vi "from string.vi"(8 "error in":errorcluster, 9 "data":string, 10 "version":string, 11 "Profibus Module configuration in":refnum<class "Profibus Module configuration.lvclass">) -> (0 "error out":errorcluster, 3 "Profibus Module configuration out":refnum<class "Profibus Module configuration.lvclass">)   [LabVIEW 2013, in "Profibus Module configuration.lvclass"]
doc: "Provides an interface for loading a module configuration from a file or other serialized data source. It is recommended that all children of this class store data in two sets--data required for its own initialization, and any data required for parent initialization--and that each implementation uses the <b>Call Parent Method</b> primitive to de-serialize parent information. As a result, it is expected that every module configuration class calls <b>component configuration.lvclass:From String.vi</b>."
uses:
  Profibus Module configuration.lvclass
  <vilib>/NI/Tag Bus Module Framework/module configuration/TBM module configuration.lvclass
  channel/Profibus channel.lvclass
  endianness setting.ctl
  <vilib>/NI/Tag Bus Module Framework/channel/TBM channel.lvclass
  error throw specification.ctl
  slave diagnostic configuration.ctl
  <vilib>/NI/Configuration Framework/serializable configuration/NISE_CEF_serializable configuration.lvclass
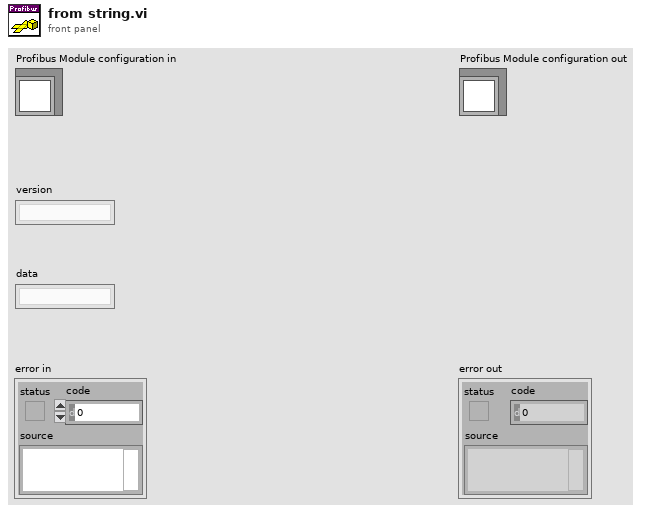
[diagram p1: front panel]
types:
  T1 = typedef "Profibus Module configuration.lvclass/slave diagnostic configuration.ctl" = cluster{"slave":i8, "report":bool, "channel":refnum<class "TBM channel.lvclass">, "error specs":T2[]}
  T2 = typedef "Profibus Module configuration.lvclass/error throw specification.ctl" = cluster{"byte":i32, "bit":i32, "inverted?":bool, "error":i32}
  T3 = typedef "Profibus Module configuration.lvclass/endianness setting.ctl" = cluster{"slave":i8, "big endian":bool}
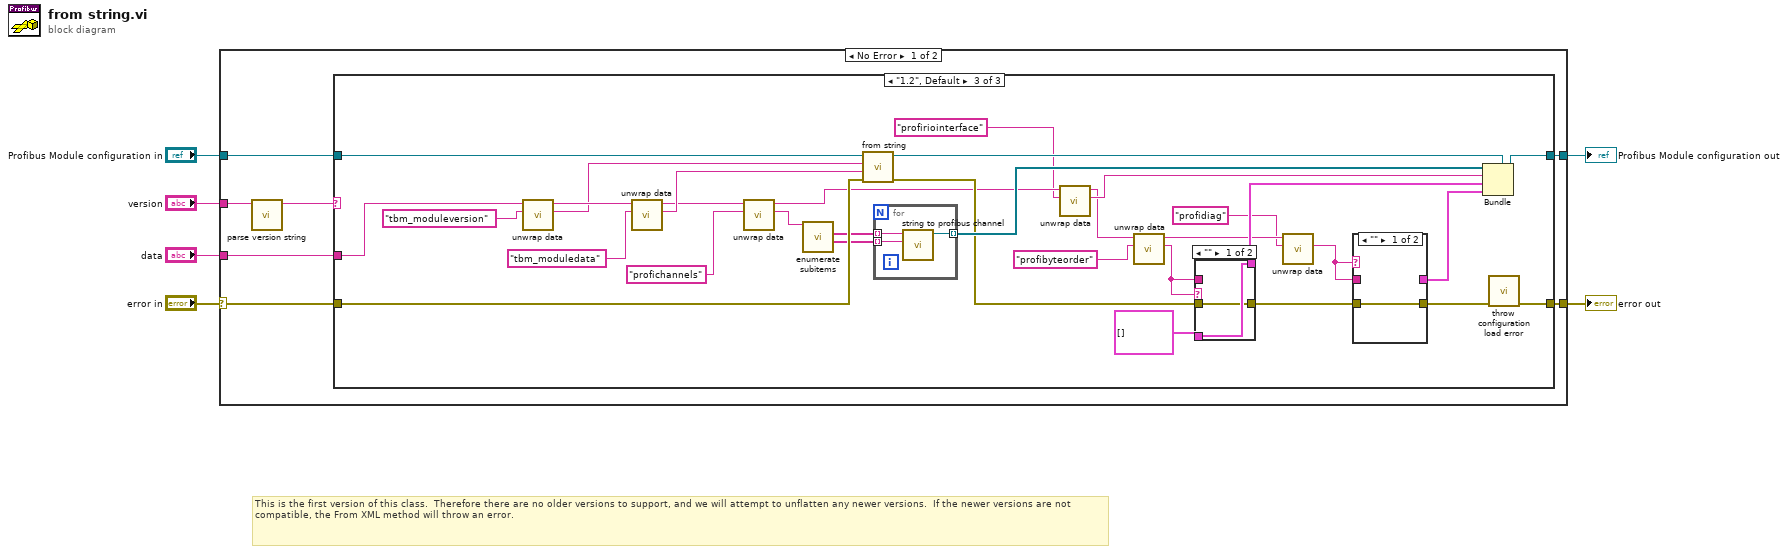
[diagram p0: block diagram]
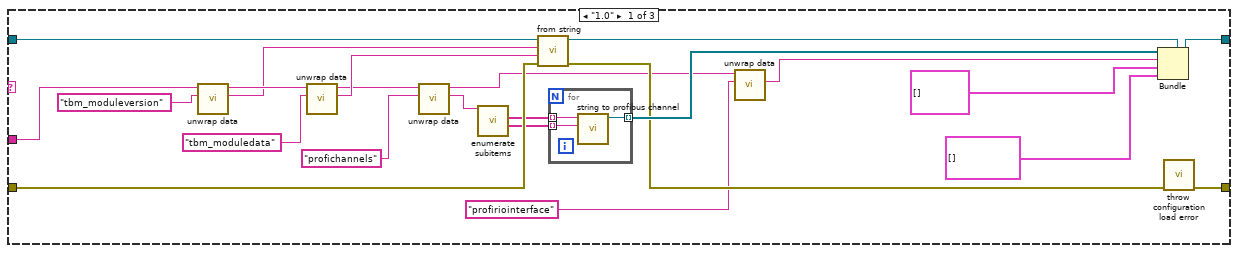
[diagram p2: hidden frame]
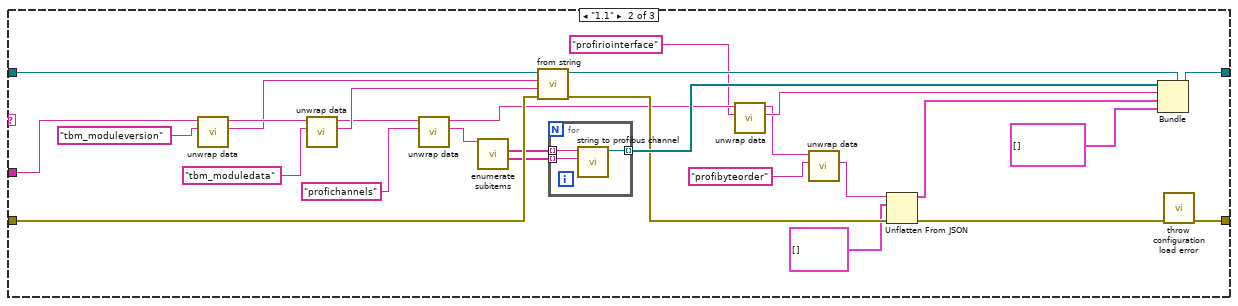
[diagram p3: hidden frame]
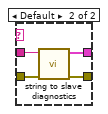
[diagram p4: hidden frame]
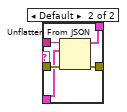
[diagram p5: hidden frame]
diagram:
  # "This is the first version of this class.  Therefore there are no older versions to support, and we will attempt to unflatten any newer versions.  If the newer versions are not compatible, the From XML method will throw an error."
  n1 = case shown="No Error" "error in" {
    selector: "error in" -> [w7 w119]
    tunnel: "data" -> [w13 _]
    tunnel: "Profibus Module configuration in" -> [w12 w118]
    tunnel: [w11 w118] -> w5
    tunnel: [w10 w119] -> w4
    tunnel: "version" -> [w9 _]
    frame No Error {
      n2 = call <vilib>:"parse version string.vi"("full version"=w9) -> ("major.minor version"=w8:string)  [unwired: 7 in, 3 out]
      n3 = case shown="\"1.2\", Default" w8 {
        tunnel: w13 -> [w32 w63 w98]
        tunnel: w7 -> [w31 w62 w97]
        tunnel: w12 -> [w36 w67 w102]
        tunnel: [w26 w57 w92] -> w11
        tunnel: [w34 w65 w100] -> w10
        frame "1.0" {
          n4 = call <vilib>:"unwrap data.vi"("identifier"="tbm_moduleversion" ("additional identifier"), "data to unwrap"=w32) -> ("unwrapped data"=w27:string, "remaining string"=w33:string)  [unwired: 8 in]
          n5 = call <vilib>:"unwrap data.vi"("identifier"="tbm_moduledata" ("additional identifier"), "data to unwrap"=w33) -> ("unwrapped data"=w29:string, "remaining string"=w25:string)  [unwired: 8 in]
          n6 = call <vilib>:"unwrap data.vi"("identifier"="profichannels" ("additional identifier"), "data to unwrap"=w25) -> ("unwrapped data"=w23:string, "remaining string"=w18:string)  [unwired: 8 in]
          n7 = call <vilib>:"enumerate subitems.vi"("data to enumerate"=w23) -> ("associated data"=w21:string[], "discovered subitems"=w22:string[])  [unwired: 8 in, 1 out]
          n8 = call-parent "from string.vi"("error in"=w31, "data"=w29, "version"=w27, "module configuration in"=w36) -> ("error out"=w19:errorcluster, "module configuration out"=w35:refnum<class "Profibus Module configuration.lvclass">)  [unwired: 6 in]
          n9 = for {
            tunnel: w22 -> [w39] mode=indexing
            tunnel: w21 -> [w38] mode=indexing
            tunnel: [w37] -> w20 mode=indexing
            n10 = call "string to profibus channel.vi"("channel data"=w38, "identifier"=w39) -> ("Profibus channel"=w37:refnum<class "Profibus channel.lvclass">)  [unwired: 9 in]
          }
          n11 = call <vilib>:"unwrap data.vi"("identifier"="profiriointerface" ("additional identifier"), "data to unwrap"=w18) -> ("unwrapped data"=w17:string)  [unwired: 8 in, 1 out]
          n12 = Bundle(cluster=w35, w20, w17, T3[] [] ("byte orders"), T1[] [] ("slave diagnostics")) -> (w26:refnum<class "Profibus Module configuration.lvclass">)
          n13 = call <vilib>:"throw configuration load error.vi"("error in"=w19) -> ("error out"=w34:errorcluster)  [unwired: 10 in]
        }
        frame "1.1" {
          n14 = call <vilib>:"unwrap data.vi"("identifier"="tbm_moduleversion" ("additional identifier"), "data to unwrap"=w63) -> ("unwrapped data"=w58:string, "remaining string"=w64:string)  [unwired: 8 in]
          n15 = call <vilib>:"unwrap data.vi"("identifier"="tbm_moduledata" ("additional identifier"), "data to unwrap"=w64) -> ("unwrapped data"=w60:string, "remaining string"=w56:string)  [unwired: 8 in]
          n16 = call <vilib>:"unwrap data.vi"("identifier"="profichannels" ("additional identifier"), "data to unwrap"=w56) -> ("unwrapped data"=w54:string, "remaining string"=w49:string)  [unwired: 8 in]
          n17 = call <vilib>:"enumerate subitems.vi"("data to enumerate"=w54) -> ("associated data"=w52:string[], "discovered subitems"=w53:string[])  [unwired: 8 in, 1 out]
          n18 = call-parent "from string.vi"("error in"=w62, "data"=w60, "version"=w58, "module configuration in"=w67) -> ("error out"=w50:errorcluster, "module configuration out"=w66:refnum<class "Profibus Module configuration.lvclass">)  [unwired: 6 in]
          n19 = for {
            tunnel: w53 -> [w70] mode=indexing
            tunnel: w52 -> [w69] mode=indexing
            tunnel: [w68] -> w51 mode=indexing
            n20 = call "string to profibus channel.vi"("channel data"=w69, "identifier"=w70) -> ("Profibus channel"=w68:refnum<class "Profibus channel.lvclass">)  [unwired: 9 in]
          }
          n21 = call <vilib>:"unwrap data.vi"("identifier"="profiriointerface" ("additional identifier"), "data to unwrap"=w49) -> ("unwrapped data"=w48:string, "remaining string"=w46:string)  [unwired: 8 in]
          n22 = call <vilib>:"unwrap data.vi"("identifier"="profibyteorder" ("additional identifier"), "data to unwrap"=w46) -> ("unwrapped data"=w44:string)  [unwired: 8 in, 1 out]
          n23 = Unflatten From JSON(JSON string=w44, type and defaults=T3[] [] ("byte orders"), error in (no error)=w50) -> (value=w42:T3[], error out=w41:errorcluster)  [unwired: 4 in]
          n24 = Bundle(cluster=w66, w51, w48, w42, T1[] [] ("slave diagnostics")) -> (w57:refnum<class "Profibus Module configuration.lvclass">)
          n25 = call <vilib>:"throw configuration load error.vi"("error in"=w41) -> ("error out"=w65:errorcluster)  [unwired: 10 in]
        }
        frame "1.2", Default {
          n26 = call <vilib>:"unwrap data.vi"("identifier"="tbm_moduleversion" ("additional identifier"), "data to unwrap"=w98) -> ("unwrapped data"=w93:string, "remaining string"=w99:string)  [unwired: 8 in]
          n27 = call <vilib>:"unwrap data.vi"("identifier"="tbm_moduledata" ("additional identifier"), "data to unwrap"=w99) -> ("unwrapped data"=w95:string, "remaining string"=w91:string)  [unwired: 8 in]
          n28 = call <vilib>:"unwrap data.vi"("identifier"="profichannels" ("additional identifier"), "data to unwrap"=w91) -> ("unwrapped data"=w89:string, "remaining string"=w84:string)  [unwired: 8 in]
          n29 = call <vilib>:"enumerate subitems.vi"("data to enumerate"=w89) -> ("associated data"=w87:string[], "discovered subitems"=w88:string[])  [unwired: 8 in, 1 out]
          n30 = call-parent "from string.vi"("error in"=w97, "data"=w95, "version"=w93, "module configuration in"=w102) -> ("error out"=w85:errorcluster, "module configuration out"=w101:refnum<class "Profibus Module configuration.lvclass">)  [unwired: 6 in]
          n31 = for {
            tunnel: w88 -> [w117] mode=indexing
            tunnel: w87 -> [w116] mode=indexing
            tunnel: [w115] -> w86 mode=indexing
            n32 = call "string to profibus channel.vi"("channel data"=w116, "identifier"=w117) -> ("Profibus channel"=w115:refnum<class "Profibus channel.lvclass">)  [unwired: 9 in]
          }
          n33 = call <vilib>:"unwrap data.vi"("identifier"="profiriointerface" ("additional identifier"), "data to unwrap"=w84) -> ("unwrapped data"=w83:string, "remaining string"=w81:string)  [unwired: 8 in]
          n34 = call <vilib>:"unwrap data.vi"("identifier"="profibyteorder" ("additional identifier"), "data to unwrap"=w81) -> ("unwrapped data"=w72:string, "remaining string"=w77:string)  [unwired: 8 in]
          n35 = case shown="\"\"" w72 {
            tunnel: w85 -> [w108 w114]
            tunnel: w72 -> [_ w113]
            tunnel: T3[] [] ("byte orders") -> [w109 w112]
            tunnel: [w109 w111] -> w78
            tunnel: [w108 w110] -> w74
            frame "" {
            }
            frame Default {
              n36 = Unflatten From JSON(JSON string=w113, type and defaults=w112, error in (no error)=w114) -> (value=w111:T3[], error out=w110:errorcluster)  [unwired: 4 in]
            }
          }
          n37 = call <vilib>:"unwrap data.vi"("identifier"="profidiag", "data to unwrap"=w77) -> ("unwrapped data"=w71:string)  [unwired: 8 in, 1 out]
          n38 = case shown="\"\"" w71 {
            tunnel: w71 -> [_ w107]
            tunnel: [_ w106] -> w75
            tunnel: w74 -> [w103 w105]
            tunnel: [w103 w104] -> w73
            frame "" {
            }
            frame Default {
              n39 = call "string to slave diagnostics.vi"("error in"=w105, "data string"=w107) -> ("error out"=w104:errorcluster, "slave diagnostics"=w106:T1[])  [unwired: 8 in]
            }
          }
          n40 = Bundle(cluster=w101, w86, w83, w78, w75) -> (w92:refnum<class "Profibus Module configuration.lvclass">)
          n41 = call <vilib>:"throw configuration load error.vi"("error in"=w73) -> ("error out"=w100:errorcluster)  [unwired: 10 in]
        }
      }
    }
    frame Error {
    }
  }
  "error out" <- w4
  "Profibus Module configuration out" <- w5
